vi "python.vi"() -> ()   [LabVIEW 2017]
panel:
  in  "stop":bool
  out "Sum":dbl
  in  "Input 2":dbl
  in  "Input 1":dbl
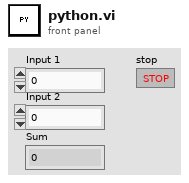
[diagram p1: front panel]
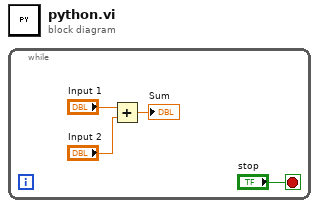
[diagram p0: block diagram]
diagram:
  n1 = while {
    stop <- "stop" stop-if-true
    n2 = Add(x="Input 1", y="Input 2") -> (x+y=→"Sum":dbl)
  }
